vi "Example Button Callback - ButtonPressed Callback.vi"(4 "ButtonPressed":refnum<user-event>, 5 "Event Data":cluster{"sender":refnum<k24>, "button":u8}, 6 "Control Ref":refnum<k24>, 7 "Event Common Data":T1) -> ()   [LabVIEW 2013]
uses:
  C:/tf/play/labview/Tinkerforge.dll
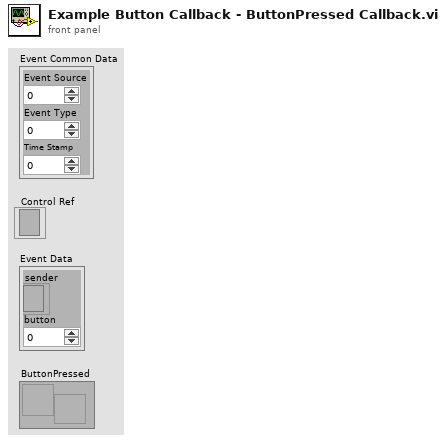
[diagram p1: front panel]
types:
  T1 = cluster{"Event Source":i32, "Event Type":u32, "Time Stamp":u32}
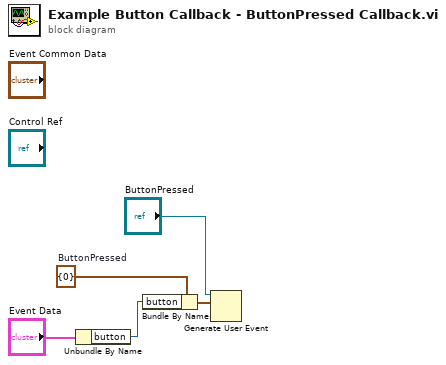
[diagram p0: block diagram]
diagram:
  w4 = cluster{"button":u8} {"button"=0}  # ButtonPressed
  n1 = Unbundle By Name("Event Data") -> ("button"=w2:u8)
  n2 = Bundle By Name(cluster=w4, "button"=w2) -> (w5:cluster{"button":u8})
  n3 = Generate User Event(user event="ButtonPressed", event data cluster=w5) -> ()  [unwired: 2 in, 2 out]
